vi "AckermannADSLabviewExample.vi"() -> ()   [LabVIEW 2020]
uses:
  <instrlib>/_Ackermann Automation/TwinCAT Ads Library/TcAdsLV_Common/TypeDefs/ClusterAdsSymbolEntry.ctl
  <instrlib>/_Ackermann Automation/TwinCAT Ads Library/TcAdsLV_Common/TypeDefs/EnumDatatypeTc.ctl
  <instrlib>/_Ackermann Automation/TwinCAT Ads Library/TcAdsLV_Common/TypeDefs/ClusterWriteData.ctl
  <instrlib>/_Ackermann Automation/TwinCAT Ads Library/TcAdsLV_Common/TypeDefs/ClusterRegistersAddress.ctl
  <instrlib>/_Ackermann Automation/TwinCAT Ads Library/TcAdsLV_Common/TypeDefs/ClusterReadDataAddress.ctl
  <instrlib>/_Ackermann Automation/TwinCAT Ads Library/TcAdsLV_Common/TypeDefs/ClusterWriteDataAddress.ctl
  <instrlib>/_Ackermann Automation/TwinCAT Ads Library/TcAdsLV_Common/TypeDefs/EnumAdsStates.ctl
  <instrlib>/_Ackermann Automation/TwinCAT Ads Library/TcAdsLV_Common/TypeDefs/ClusterVersionInfo.ctl
  <instrlib>/_Ackermann Automation/TwinCAT Ads Library/TcAdsLV_Common/TypeDefs/ClusterReadData.ctl
  <instrlib>/_Ackermann Automation/TwinCAT Ads Library/TcAdsLV_Common/TypeDefs/EnumControlAdsState.ctl
  <instrlib>/_Ackermann Automation/TwinCAT Ads Library/TcAdsLV_Dll/Functions/ReadSymbolByNameVariant.vi
  <instrlib>/_Ackermann Automation/TwinCAT Ads Library/TcAdsLV_Dll/Functions/WriteSymbolByNameArrayU8.vi
  <instrlib>/_Ackermann Automation/TwinCAT Ads Library/TcAdsLV_Dll/TcAdsLV_Dll_3.lvlib
  <instrlib>/_Ackermann Automation/TwinCAT Ads Library/TcAdsLV_Common/TcAdsLV_Common_3.lvlib
panel:
  out "Device Name":string
  out "Version":T1
  out "Device State":T2=enum."IDLE"
  out "ADS State":T2=enum."IDLE"
  out "Write Errors 2":errorcluster[](array[cluster])
  out "Execution Time ms 4":i32
  in  "Write Data 3":T3[](array[typedef]) {"Index Offset" format="%.0x"; "Index Group" format="%.0x"}
  out "Execution Time ms 3":i32
  in  "IndexGroup 2":u32 format="%x"
  in  "IndexOffset 2":u32 format="%x"
  in  "Write Data 2":u8[](array[numeric])
  out "Execution Time ms 2":i32
  out "Read Data 2":T4[](array[typedef]) {"Index Offset" format="%.0x"; "Index Group" format="%.0x"}
  in  "Registers Addresses":T5[](array[typedef]) {"Index Offset" format="%.0x"; "Index Group" format="%.0x"}
  in  "IndexGroup":u32 format="%x"
  in  "IndexOffset":u32 format="%x"
  out "Bytes Read":u32
  out "Read Data":u8[](array[numeric])
  out "Execution Time ms":i32
  in  "Length":u32=4
  out "Execution Time ms 7":i32
  out "Write Errors":errorcluster[](array[cluster])
  in  "Write Data":T6[](array[typedef])
  in  "Names":string[](array[string])
  out "Execution Time ms 6":i32
  out "Read Data 3":T7[](array[typedef])
  out "Execution Time ms 5":i32
  in  "Data 2":u8[](array[numeric])
  in  "Name 2":string
  out "Execution Time ms 8":i32
  out "Data":variant
  out "Count":u32
  out "Data Type":T8
  in  "Name":string
  in  "Query Symbols":bool=TRUE
  out "Symbols Found":bool
  out "Symbols":T9[](array[typedef]) {"Index Offset" format="%.0x"; "Index Group" format="%.0x"}
  in  "NetId":string="192.168.2.100.1.1"
  in  "Target Port":u16=801
  out "Activated Version":i32
  out "Activation Ok":bool
  in  "License Number":string="00000000"
  in  "ADS State 2":T10
  out "error out":errorcluster
  in  "error in":errorcluster
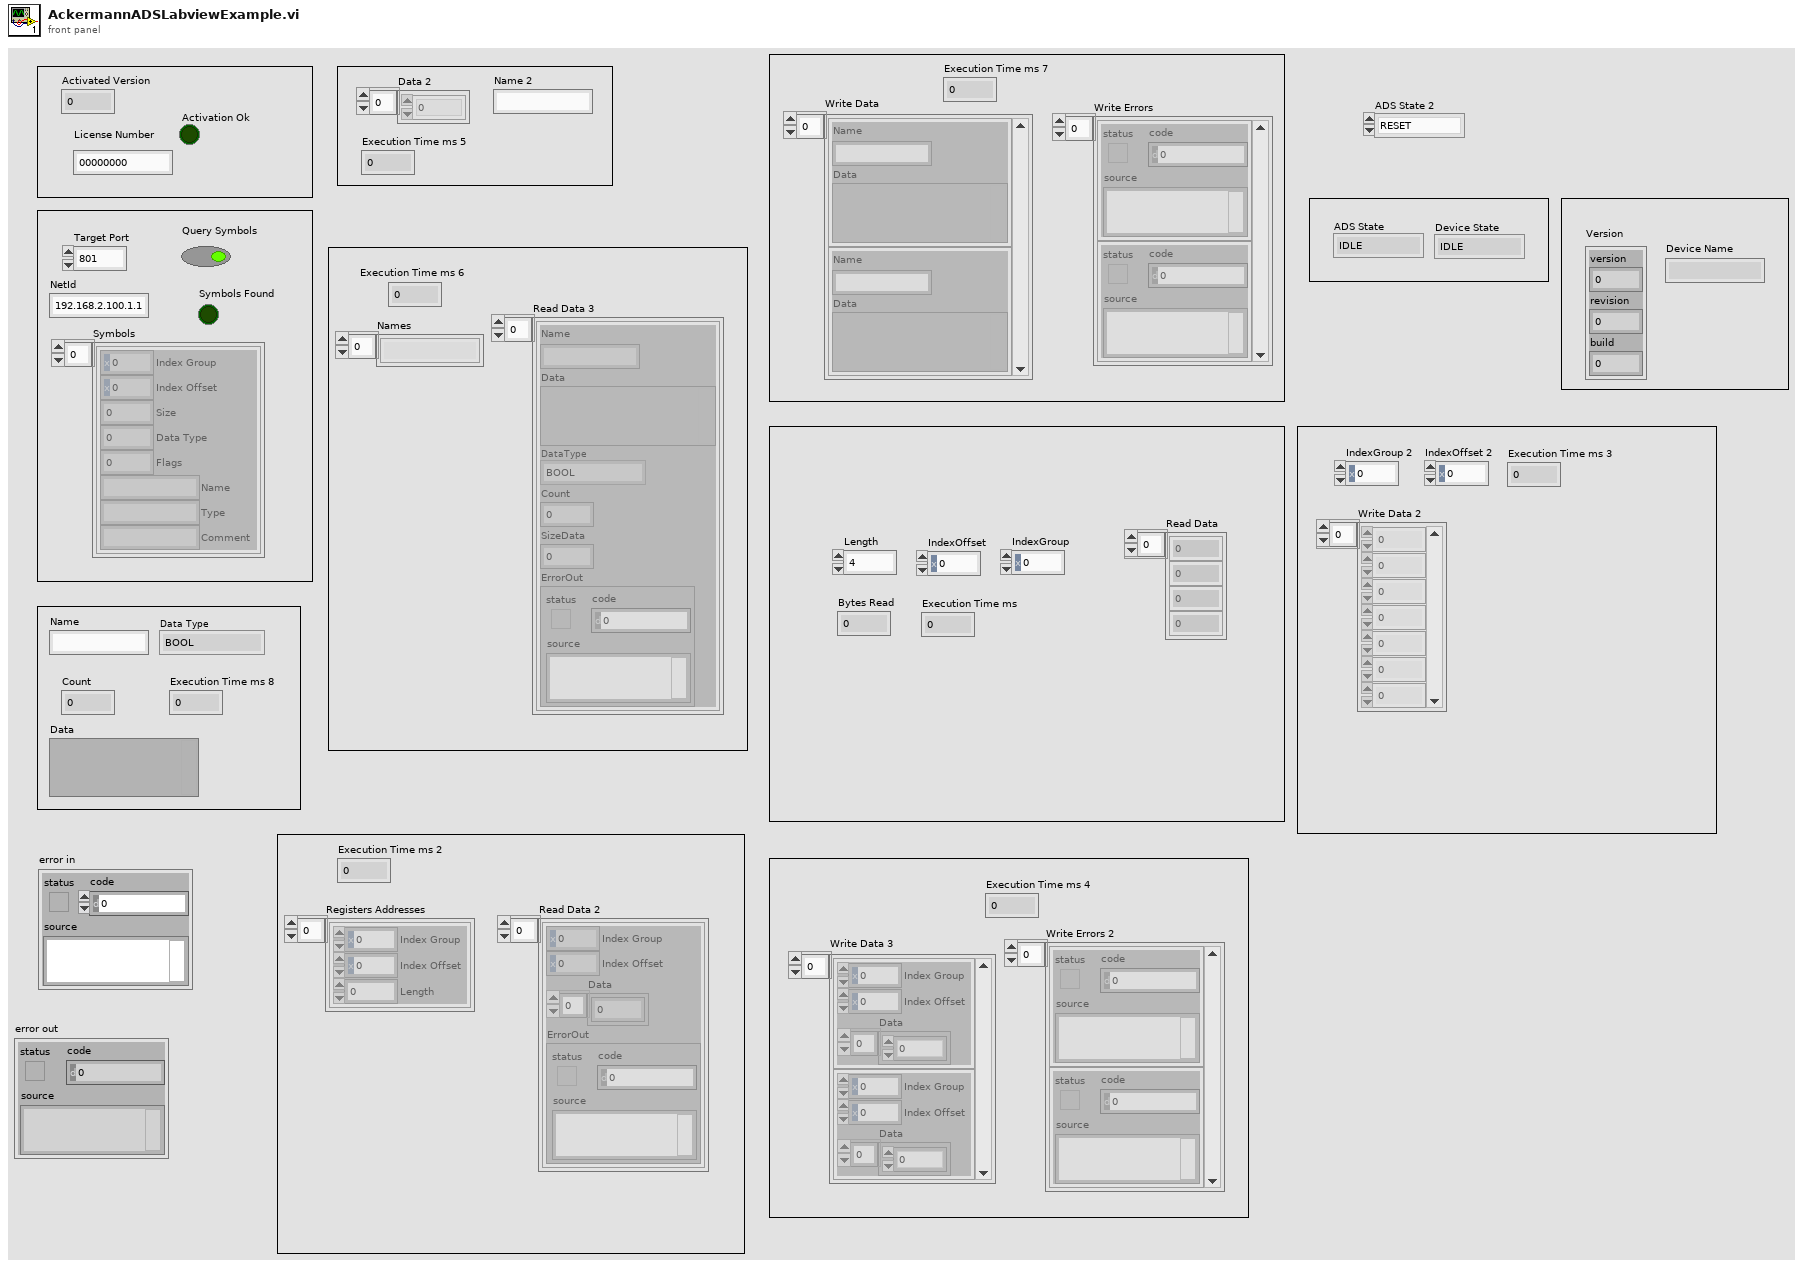
[diagram p1: front panel]
types:
  T1 = typedef "TcAdsLV_Common_3.lvlib/ClusterVersionInfo.ctl" = cluster{"version":u8, "revision":u8, "build":u16}
  T2 = typedef "TcAdsLV_Common_3.lvlib/EnumAdsStates.ctl" = enum16{"INVALID", "IDLE", "RESET", "INIT", "START", "RUN", "STOP", "SAVECFG", "LOADCFG", "POWERFAILURE", "POWERGOOD", "ERROR", "SHUTDOWN", "SUSPEND", "RESUME", "CONFIG", "RECONFIG", "STOPPING", "INCOMPATIBLE", "EXCEPTION"}
  T3 = typedef "TcAdsLV_Common_3.lvlib/ClusterWriteDataAddress.ctl" = cluster{"Index Group":u32, "Index Offset":u32, "Data":u8[]}
  T4 = typedef "TcAdsLV_Common_3.lvlib/ClusterReadDataAddress.ctl" = cluster{"Index Group":u32, "Index Offset":u32, "Data":u8[], "ErrorOut":errorcluster}
  T5 = typedef "TcAdsLV_Common_3.lvlib/ClusterRegistersAddress.ctl" = cluster{"Index Group":u32, "Index Offset":u32, "Length":u32}
  T6 = typedef "TcAdsLV_Common_3.lvlib/ClusterWriteData.ctl" = cluster{"Name":string, "Data":variant}
  T7 = typedef "TcAdsLV_Common_3.lvlib/ClusterReadData.ctl" = cluster{"Name":string, "Data":variant, "DataType":T8, "Count":u32, "SizeData":u32, "ErrorOut":errorcluster}
  T8 = typedef "TcAdsLV_Common_3.lvlib/EnumDatatypeTc.ctl" = enum16{"BOOL", "BYTE", "WORD", "DWORD", "SINT", "USINT", "INT", "UINT", "DINT", "UDINT", "LINT", "ULINT", "REAL", "LREAL", "STRING", "TIME", "TOD", "DATE", "DT", "FLEXIBLE"}
  T9 = typedef "TcAdsLV_Common_3.lvlib/ClusterAdsSymbolEntry.ctl" = cluster{"Index Group":u32, "Index Offset":u32, "Size":u32, "Data Type":u32, "Flags":u32, "Name":string, "Type":string, "Comment":string}
  T10 = typedef "TcAdsLV_Common_3.lvlib/EnumControlAdsState.ctl" = enum16{"RESET", "RUN", "STOP", "SAVECFG"}
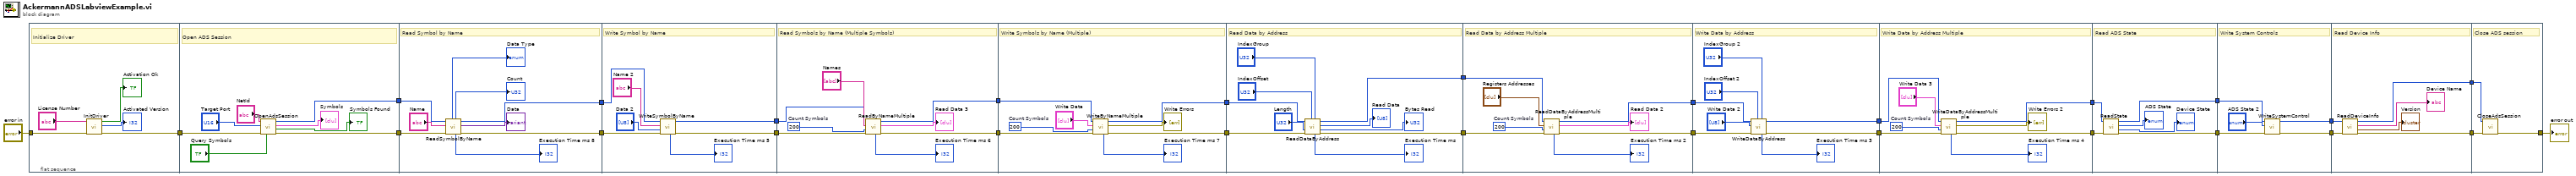
[diagram p0: block diagram]
diagram:
  n1 = flat-sequence {
    tunnel: "error in" -> [w29]
    tunnel: [w28] -> w20
    tunnel: w20 -> [w35]
    tunnel: [w34] -> w19
    tunnel: [w33] -> w8
    tunnel: w19 -> [w45]
    tunnel: [w44] -> w18
    tunnel: w8 -> [w43]
    tunnel: [w42] -> w7
    tunnel: w18 -> [w53]
    tunnel: [w52] -> w17
    tunnel: w7 -> [w51]
    tunnel: [w50] -> w6
    tunnel: w17 -> [w61]
    tunnel: [w60] -> w16
    tunnel: w6 -> [w58]
    tunnel: [w57] -> w5
    tunnel: w16 -> [w69]
    tunnel: [w68] -> w15
    tunnel: w5 -> [w66]
    tunnel: [w65] -> w4
    tunnel: w15 -> [w76]
    tunnel: [w75] -> w14
    tunnel: w4 -> [w74]
    tunnel: [w73] -> w3
    tunnel: w14 -> [w86]
    tunnel: [w85] -> w13
    tunnel: w3 -> [w84]
    tunnel: [w83] -> w2
    tunnel: w13 -> [w94]
    tunnel: [w93] -> w12
    tunnel: w2 -> [w92]
    tunnel: [w91] -> w1
    tunnel: [w102] -> w26
    tunnel: w12 -> [w101]
    tunnel: [w100] -> w9
    tunnel: w1 -> [w99]
    tunnel: w26 -> [w110]
    tunnel: [w109] -> w25
    tunnel: [w108] -> w24
    tunnel: w9 -> [w107]
    tunnel: w25 -> [w116]
    tunnel: w24 -> [w115]
    tunnel: [w114] -> w23
    tunnel: [w113] -> w11
    tunnel: w23 -> [w122]
    tunnel: [w121] -> w22
    tunnel: w11 -> [w120]
    tunnel: [w119] -> w10
    tunnel: w22 -> [w126]
    tunnel: [w125] -> w21
    tunnel: w10 -> [w124]
    frame #0 {
      # "Initialize Driver"
      n2 = call <instrlib>:"InitDriver.vi"("error in"=w29, "License Number"="License Number") -> ("error out"=w28:errorcluster, "Activated Version"=→"Activated Version":i32, "Activation Ok"=→"Activation Ok":bool)  [unwired: 7 in]
    }
    frame #1 {
      # "Open ADS Session"
      n3 = call <instrlib>:"OpenAdsSession.vi"("Query Symbols"="Query Symbols", "error in"=w35, "Target Port"="Target Port", "NetId"="NetId") -> ("error out"=w34:errorcluster, "Symbols Found"=→"Symbols Found":bool, "Symbols"=→"Symbols":T9[], "Session Ref"=w33:u32)  [unwired: 4 in]
    }
    frame #2 {
      # "Read Symbol by Name"
      n4 = call-poly <instrlib>:"ReadSymbolByName.vi"("error in"=w45, "Name"="Name", "Session Ref"=w43) -> ("error out"=w44:errorcluster, "Data"=→"Data":variant, "Session Ref out"=w42:u32, "Execution Time ms"=→"Execution Time ms 8":i32, "Count"=→"Count":u32, "Data Type"=→"Data Type":T8)  [unwired: 2 in, 1 out]
    }
    frame #3 {
      # "Write Symbol by Name"
      n5 = call-poly <instrlib>:"WriteSymbolByName.vi"("error in"=w53, "Data"="Data 2", "Name"="Name 2", "Session Ref"=w51) -> ("error out"=w52:errorcluster, "Session Ref out"=w50:u32, "Execution Time ms"=→"Execution Time ms 5":i32)  [unwired: 5 in]
    }
    frame #4 {
      w59 = 200  # Count Symbols
      # "Read Symbols by Name (Multiple Symbols)"
      n6 = call <instrlib>:"ReadByNameMultiple.vi"("error in"=w61, "Count Symbols"=w59, "Names"="Names", "Session Ref"=w58) -> ("error out"=w60:errorcluster, "Read Data"=→"Read Data 3":T7[], "Session Ref out"=w57:u32, "Execution Time ms"=→"Execution Time ms 6":i32)  [unwired: 4 in]
    }
    frame #5 {
      w67 = 200  # Count Symbols
      # "Write Symbols by Name (Multiple)"
      n7 = call <instrlib>:"WriteByNameMultiple.vi"("error in"=w69, "Count Symbols"=w67, "Write Data"="Write Data", "Session Ref"=w66) -> ("error out"=w68:errorcluster, "Write Errors"=→"Write Errors":errorcluster[], "Session Ref out"=w65:u32, "Execution Time ms"=→"Execution Time ms 7":i32)  [unwired: 4 in]
    }
    frame #6 {
      # "Read Data by Address"
      n8 = call <instrlib>:"ReadDataByAddress.vi"("IndexGroup"="IndexGroup", "IndexOffset"="IndexOffset", "error in"=w76, "Length"="Length", "Session Ref"=w74) -> ("error out"=w75:errorcluster, "Bytes Read"=→"Bytes Read":u32, "Read Data"=→"Read Data":u8[], "Session Ref out"=w73:u32, "Execution Time ms"=→"Execution Time ms":i32)  [unwired: 2 in]
    }
    frame #7 {
      w87 = 200  # Count Symbols
      # "Read Data by Address Multiple"
      n9 = call <instrlib>:"ReadDataByAddressMultiple.vi"("error in"=w86, "Count Symbols"=w87, "Registers Addresses"="Registers Addresses", "Session Ref"=w84) -> ("error out"=w85:errorcluster, "Read Data"=→"Read Data 2":T4[], "Session Ref out"=w83:u32, "Execution Time ms"=→"Execution Time ms 2":i32)  [unwired: 4 in]
    }
    frame #8 {
      # "Write Data by Address"
      n10 = call <instrlib>:"WriteDataByAddress.vi"("IndexGroup"="IndexGroup 2", "IndexOffset"="IndexOffset 2", "error in"=w94, "Write Data"="Write Data 2", "Session Ref"=w92) -> ("error out"=w93:errorcluster, "Session Ref out"=w91:u32, "Execution Time ms"=→"Execution Time ms 3":i32)  [unwired: 4 in]
    }
    frame #9 {
      w103 = 200  # Count Symbols
      # "Write Data by Address Multiple"
      n11 = call <instrlib>:"WriteDataByAddressMultiple.vi"("error in"=w101, "Count Symbols"=w103, "Write Data"="Write Data 3", "Session Ref"=w99) -> ("error out"=w102:errorcluster, "Write Errors"=→"Write Errors 2":errorcluster[], "Session Ref out"=w100:u32, "Execution Time ms"=→"Execution Time ms 4":i32)  [unwired: 4 in]
    }
    frame #10 {
      # "Read ADS State"
      n12 = call <instrlib>:"ReadState.vi"("error in"=w110, "Session Ref"=w107) -> ("error out"=w109:errorcluster, "Device State"=→"Device State":T2, "ADS State"=→"ADS State":T2, "Session Ref out"=w108:u32)  [unwired: 6 in]
    }
    frame #11 {
      # "Write System Controls"
      n13 = call <instrlib>:"WriteSystemControl.vi"("error in"=w116, "ADS State"="ADS State 2", "Session Ref"=w115) -> ("error out"=w114:errorcluster, "Session Ref out"=w113:u32)  [unwired: 7 in]
    }
    frame #12 {
      # "Read Device Info"
      n14 = call <instrlib>:"ReadDeviceInfo.vi"("error in"=w122, "Session Ref"=w120) -> ("error out"=w121:errorcluster, "Version"=→"Version":T1, "Device Name"=→"Device Name":string, "Session Ref out"=w119:u32)  [unwired: 6 in]
    }
    frame #13 {
      # "Close ADS session"
      n15 = call <instrlib>:"CloseAdsSession.vi"("error in"=w126, "Session Ref"=w124) -> ("error out"=w125:errorcluster)  [unwired: 9 in]
    }
  }
  "error out" <- w21
